vi "Read Test Suite.vi"(11 "Test Runner in":refnum<class "Test Runner.lvclass">) -> (1 "undefined":bool, 2 "Test Suite":refnum<class "Test Suite.lvclass">, 3 "Test Runner out":refnum<class "Test Runner.lvclass">)   [LabVIEW 2020, in "Caraya.lvlib" / "Test Runner.lvclass"]
uses:
  Test Runner.lvclass
  Test Suite/Test Suite.lvclass
  Test Runner.lvclass/Test Runner.ctl
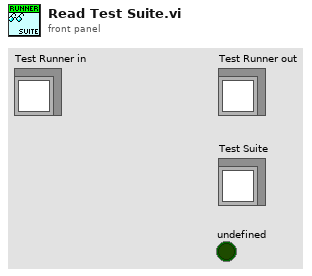
[diagram p1: front panel]
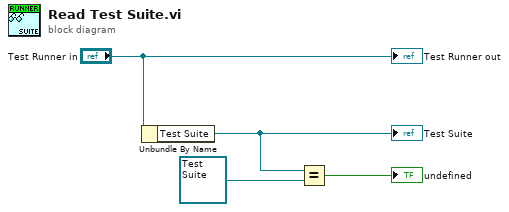
[diagram p0: block diagram]
diagram:
  n1 = Unbundle By Name("Test Runner in") -> ("Test Suite"=w3:refnum<class "Test Suite.lvclass">)
  "Test Suite" <- w3
  n2 = Equal?(x=w3, y=refnum<class "Test Suite.lvclass"> refnum) -> (x = y?=→"undefined":bool)
  "Test Runner out" <- "Test Runner in"
